vi "Create Gaussian.vi"(6 "Std. Deviation":sgl, 9 "Gaussian Filter X Size":u32, 10 "Gaussian Filter Y Size":u32, 11 "Gaussian Filter Z Size":u32) -> (2 "Array 2":sgl[][][](array[numeric]), 3 "Array":sgl[][][](array[numeric]))   [LabVIEW 2012, in "OpenCLV x64.lvlib"]
uses:
  OpenCLV x64.lvlib
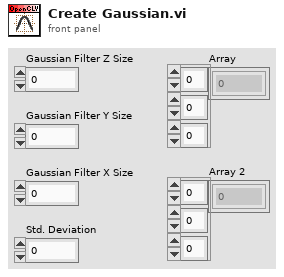
[diagram p1: front panel]
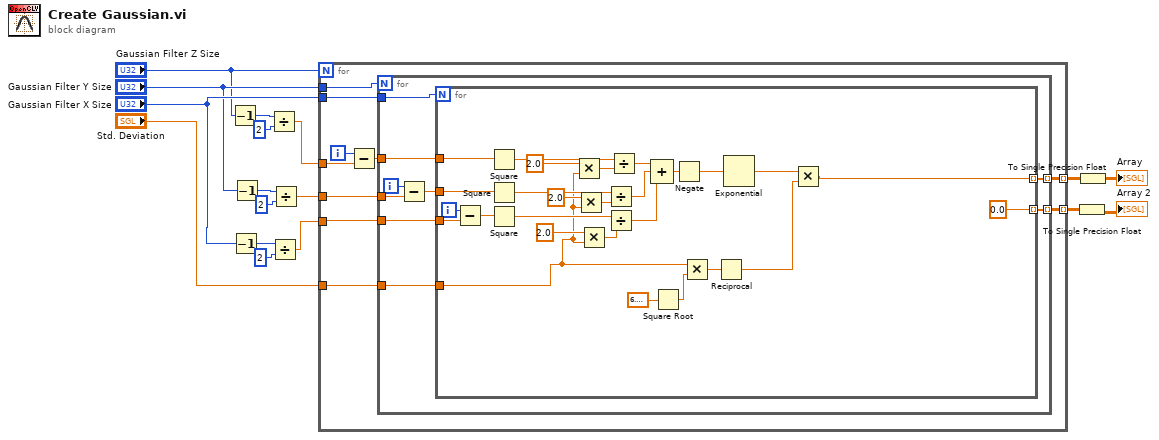
[diagram p0: block diagram]
diagram:
  n1 = Decrement(x="Gaussian Filter Z Size") -> (x-1=w4:u32)
  n2 = Decrement(x="Gaussian Filter X Size") -> (x-1=w14:u32)
  n3 = Decrement(x="Gaussian Filter Y Size") -> (x-1=w12:u32)
  n4 = Divide(x=w4, y=2) -> (x/y=w7:dbl)
  n5 = Divide(x=w14, y=2) -> (x/y=w13:dbl)
  n6 = Divide(x=w12, y=2) -> (x/y=w11:dbl)
  n7 = for {
    N: "Gaussian Filter Z Size" -> [_]
    tunnel: w7 -> [w26]
    tunnel: w11 -> [w24]
    tunnel: w13 -> [w23]
    tunnel: [w22] -> w2 mode=indexing
    tunnel: [w21] -> w3 mode=indexing
    tunnel: "Std. Deviation" -> [w20]
    tunnel: "Gaussian Filter Y Size" -> [w19]
    tunnel: "Gaussian Filter X Size" -> [w18]
    i -> [w27]
    n8 = Subtract(x=w27, y=w26) -> (x-y=w25:dbl)
    n9 = for {
      N: w19 -> [_]
      tunnel: w25 -> [w32]
      tunnel: w24 -> [w35]
      tunnel: w23 -> [w33]
      tunnel: [w31] -> w22 mode=indexing
      tunnel: [w30] -> w21 mode=indexing
      tunnel: w20 -> [w29]
      tunnel: w18 -> [w28]
      i -> [w36]
      n10 = Subtract(x=w36, y=w35) -> (x-y=w34:dbl)
      n11 = for {
        N: w28 -> [_]
        tunnel: w34 -> [w60]
        tunnel: w33 -> [w62]
        tunnel: w32 -> [w59]
        tunnel: [w39] -> w31 mode=indexing
        tunnel: [0.0 ("x")] -> w30 mode=indexing
        tunnel: w29 -> [w37]
        i -> [w63]
        n12 = Subtract(x=w63, y=w62) -> (x-y=w61:dbl)
        n13 = Square(x=w59) -> (x^2=w57:dbl)
        n14 = Square(x=w60) -> (x^2=w56:dbl)
        n15 = Square(x=w61) -> (x^2=w55:dbl)
        n16 = Multiply(x=2.0, y=w37) -> (x*y=w54:dbl)
        n17 = Multiply(x=2.0, y=w37) -> (x*y=w53:dbl)
        n18 = Multiply(x=2.0, y=w37) -> (x*y=w52:dbl)
        n19 = Divide(x=w56, y=w53) -> (x/y=w47:dbl)
        n20 = Divide(x=w55, y=w52) -> (x/y=w46:dbl)
        n21 = Divide(x=w57, y=w54) -> (x/y=w48:dbl)
        n22 = Compound Arithmetic op=ADD(w48, w47, w46) -> (w58:dbl)
        n23 = Square Root(x=6.283185307179586) -> (sqrt(x)=w42:dbl)
        n24 = Negate(x=w58) -> (-x=w45:dbl)
        n25 = Multiply(x=w37, y=w42) -> (x*y=w41:dbl)
        n26 = Reciprocal(x=w41) -> (1/x=w40:dbl)
        n27 = Exponential(1:w45) -> (0:w44:dbl)
        n28 = Multiply(x=w44, y=w40) -> (x*y=w39:dbl)
      }
    }
  }
  n29 = To Single Precision Float(number=w3) -> (single precision float=→"Array 2":sgl[][][])
  n30 = To Single Precision Float(number=w2) -> (single precision float=→"Array":sgl[][][])
